vi "求斜率k的子程序.vi"(1 "x1":dbl, 2 "x2":dbl, 3 "y1":dbl, 4 "y2":dbl) -> (0 "k":dbl)   [LabVIEW 2010]
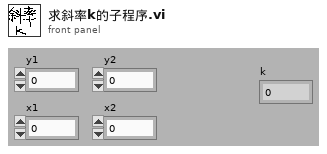
[diagram p1: front panel]
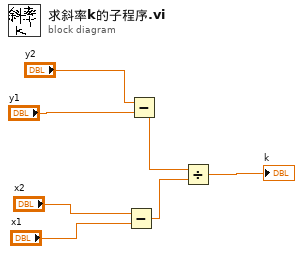
[diagram p0: block diagram]
diagram:
  n1 = Subtract(x="x2", y="x1") -> (x-y=w2:dbl)
  n2 = Subtract(x="y2", y="y1") -> (x-y=w3:dbl)
  n3 = Divide(x=w3, y=w2) -> (x/y=→"k":dbl)
